vi "1_termometro.vi"(0 "Kelvin to Fahrenheit":bool) -> (1 "Waveform Chart":dbl(graph), 2 "Celsius":dbl(slide) scale=0.0..100.0 scale format="%.2f", 3 "Fahrenheit":dbl(slide) scale=0.0..250.0 scale format="%.2f", 4 "Kelvin":dbl(slide) scale=0.0..500.0 scale format="%.2f")   [LabVIEW 2017]
panel:
  out "Celsius":string
  out "Kelvin":string
  out "Fahrenheit":string
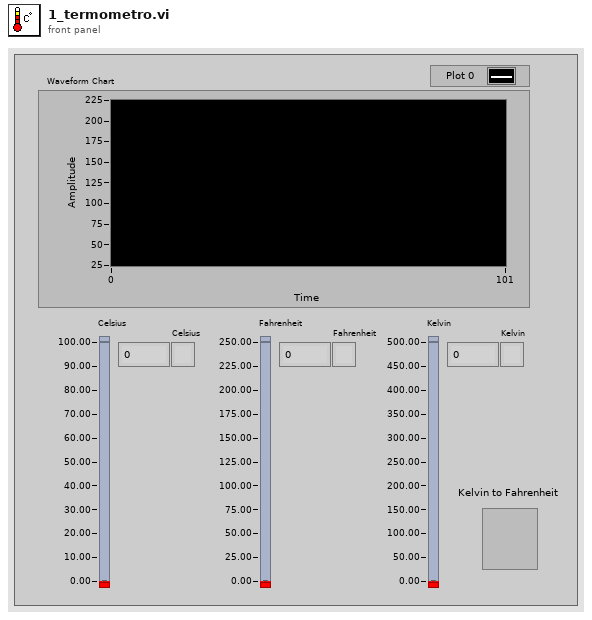
[diagram p1: front panel]
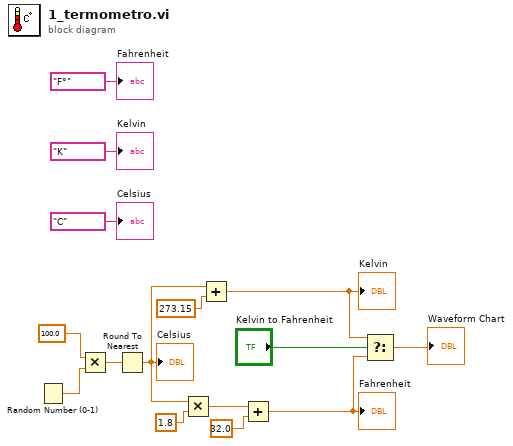
[diagram p0: block diagram]
diagram:
  n1 = Random Number (0-1)() -> (number: 0 to 1=w5:dbl)
  n2 = Multiply(x=100.0, y=w5) -> (x*y=w3:dbl)
  n3 = Round To Nearest(number=w3) -> (nearest integer value=w2:dbl)
  "Celsius" <- w2
  n4 = Multiply(x=w2, y=1.8) -> (x*y=w14:dbl)
  n5 = Add(x=w2, y=273.15) -> (x+y=w7:dbl)
  "Kelvin" <- w7
  n6 = Add(x=w14, y=32.0) -> (x+y=w6:dbl)
  "Fahrenheit" <- w6
  n7 = Select(t=w7, s="Kelvin to Fahrenheit", f=w6) -> (s? t:f=→"Waveform Chart":dbl)
  "Fahrenheit" <- "F°"
  "Kelvin" <- "K"
  "Celsius" <- "C"
